vi "Data collection Program.vi"(10 "Current File Name":path, 11 "Average file path":path) -> ()   [LabVIEW 2011]
uses:
  <vilib>/Utility/file.llb/Read From Spreadsheet File (DBL).vi
  <vilib>/Utility/file.llb/Write To Spreadsheet File (DBL).vi
panel:
  out "Array":dbl[](array[numeric])
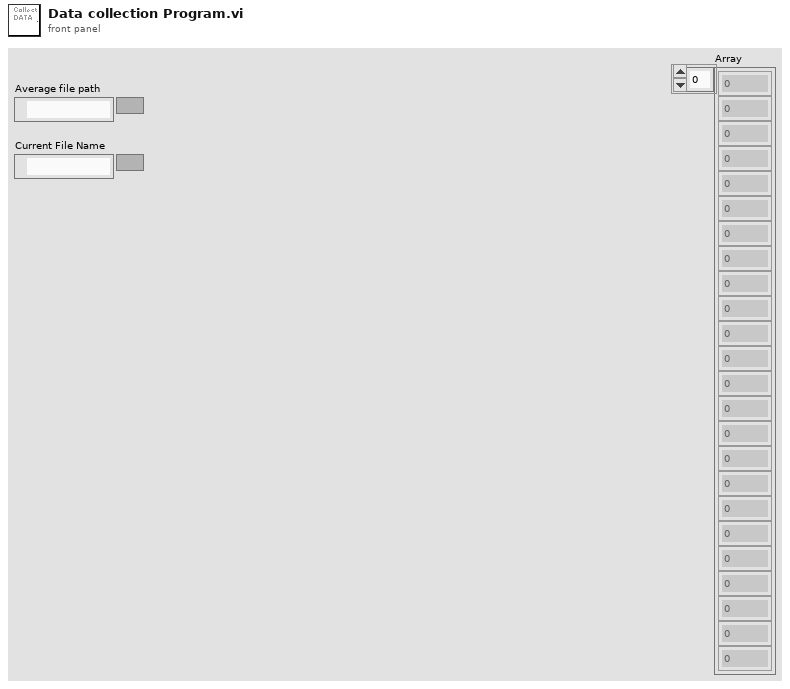
[diagram p1: front panel]
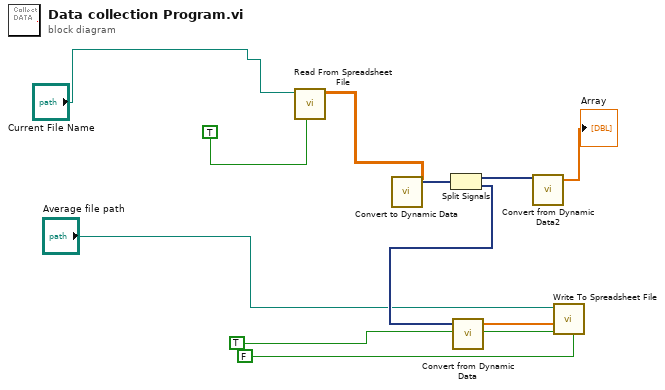
[diagram p0: block diagram]
diagram:
  n1 = call-poly <vilib>:"Read From Spreadsheet File.vi"("transpose (no:F)"=TRUE, "file path (dialog if empty)"="Current File Name") -> ("all rows"=w4:dbl[][])  [unwired: 5 in, 4 out]
  n2 = call "Convert to Dynamic Data"("2D Array"=w4) -> ("Dynamic Data Type"=w5:dynamicdata)  [unwired: 3 in]
  n3 = Split Signals(w5) -> (w2:dynamicdata, w9:dynamicdata)  [unwired: 2 in]
  n4 = call "Convert from Dynamic Data"("Dynamic Data Type"=w9) -> ("Array"=w10:dbl[])  [unwired: 3 in]
  n5 = call "Convert from Dynamic Data2"("Dynamic Data Type"=w2) -> ("Array"=→"Array":dbl[])  [unwired: 3 in]
  n6 = call-poly <vilib>:"Write To Spreadsheet File.vi"("transpose? (no:F)"=FALSE, "append to file? (new file:F)"=TRUE, "1D data"=w10, "file path (dialog if empty)"="Average file path") -> ()  [unwired: 4 in, 1 out]
